vi "Actor Core.vi"(8 "error in":errorcluster, 11 "PW3390 in":refnum<class "PW3390.lvclass">) -> (0 "error out":errorcluster, 3 "Actor out":refnum<class "Actor.lvclass">)   [LabVIEW 2024, in "PW3390 Actor.lvlib" / "PW3390.lvclass"]
doc: "<p>(<strong>Filename</strong>: <span class=\"dnl\">Actor Framework.lvlib:Actor.lvclass:Actor Core.vi</span>)</p>\n<p>Receives messages to the actor, reacts to them, and initiates any error handling that may shut the actor down.</p>\n<p>Descendant classes may override this VI to append parallel tasks for the actor to complete while it handles messages. Overrides use the <a href=\"nihelplauncher://docs/csh?context=lvcore_glang_udclass\">Call Parent Class Method</a> node.</p>"
uses:
  PW3390.lvclass
  C:/Program Files (x86)/National Instruments/LabVIEW 2024/vi.lib/ActorFramework/Actor/Actor.lvclass
  <vilib>/ActorFramework/Actor/Actor.lvclass
  <vilib>/ActorFramework/Actor/Actor.lvclass/Actor.ctl
  PW3390.lvclass/PW3390.ctl
  PW3390Func.ctl
  MFActor/ActorMessage/MF Task Name.ctl
  MFActor/NestedActorName.ctl
  MFActor/DeviceAlias.ctl
  MFActor/ActorMessage/MFActorMsg.lvclass
panel:
  out "Connected":bool
  out "MeasData":dbl[](array[numeric]) format="%.2f"
  out "UpdateData":bool
  out "In Query":bool
  out "connection ID":refnum<k5>
  out "Item":T1(array[cluster])
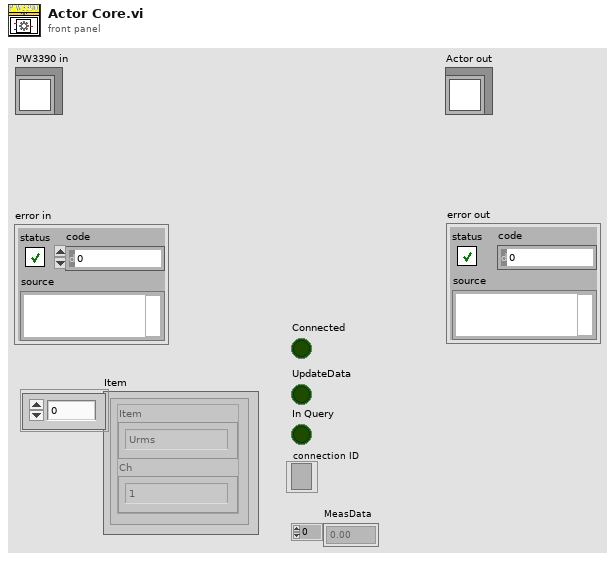
[diagram p1: front panel]
types:
  T1 = cluster{"Item":enum16{"Urms", "Umn", "Uac", "Udc", "Ufnd", "Upk+", "Upk-", "Uthd", "Urf", "Uunb", "Irms", "Imn", "Iac", "Idc", "Ifnd", "Ipk+", "Ipk-", "Ithd", "Irf", "Iunb", "P", "S", "Q", "PF", "DEG U", "DEG I", "DEG P", "f", "EFFI", "LOSS", "IH+", "IH-", "IH", "WP+", "WP-", "WP", "CH A", "CH B", "Pm", "Slip", "TEMP"}, "Ch":enum16{"1", "2", "3", "4", "12", "34", "123"}}[]
  T2 = typedef "PW3390Func.ctl" = enum16{"None", "Wiring", "Config", "Query", "ConvertData", "End"}
  T3 = cluster{"Wiring":u16, "Interface":refnum<visa-resource-name>, "1P Mode":u16, "1P CurrentLimit":dbl, "3P Mode":u16, "3P CurrentLimit":dbl}
  T4 = cluster{"DriverIn":refnum<vi>, "DriverOut":refnum<vi>}
  T5 = cluster{"ManualFetchData":refnum<vi>, "AutoFetchData":refnum<vi>, "SampleRate":refnum<vi>}
  T6 = typedef "NestedActorName.ctl" = enum16{"None", "4503#0", "4503#1", "AIO#0", "AIO#1", "DIO", "PID", "TCPIP", "TestAngle", "TestFixPt", "TestMultiPt", "TestSinWave", "PW3390"}
  T7 = typedef "MF Task Name.ctl" = enum16{"DIChanged", "UpdateErrorCode", "SetTorque", "SetDriveTorque", "DataUpdated", "RunningTestProc", "StreamCtrl", "RunPID", "StopTest", "TCP Conn", "RefreshAutoUI", "ZeroAngle", "NestedActorLaunched", "NestedActorEnded"}
  T8 = typedef "DeviceAlias.ctl" = enum16{"TQM0", "TQM1", "PM", "THERMO", "DC POWER"}
  T9 = cluster{"Data out[0]":dbl, "Data out[1]":dbl, "Data out[2]":dbl, "Data out[3]":dbl, "Data out[4]":dbl, "Data out[5]":dbl, "Data out[6]":dbl, "Data out[7]":dbl, "Data out[8]":dbl, "Data out[9]":dbl}
  T10 = cluster{"Data out[0]":dbl, "Data out[1]":dbl, "Data out[2]":dbl, "Data out[3]":dbl}
  T11 = cluster{"MF Msg Enum":T7, cluster{"MeasData":dbl[], "Device":T8}}
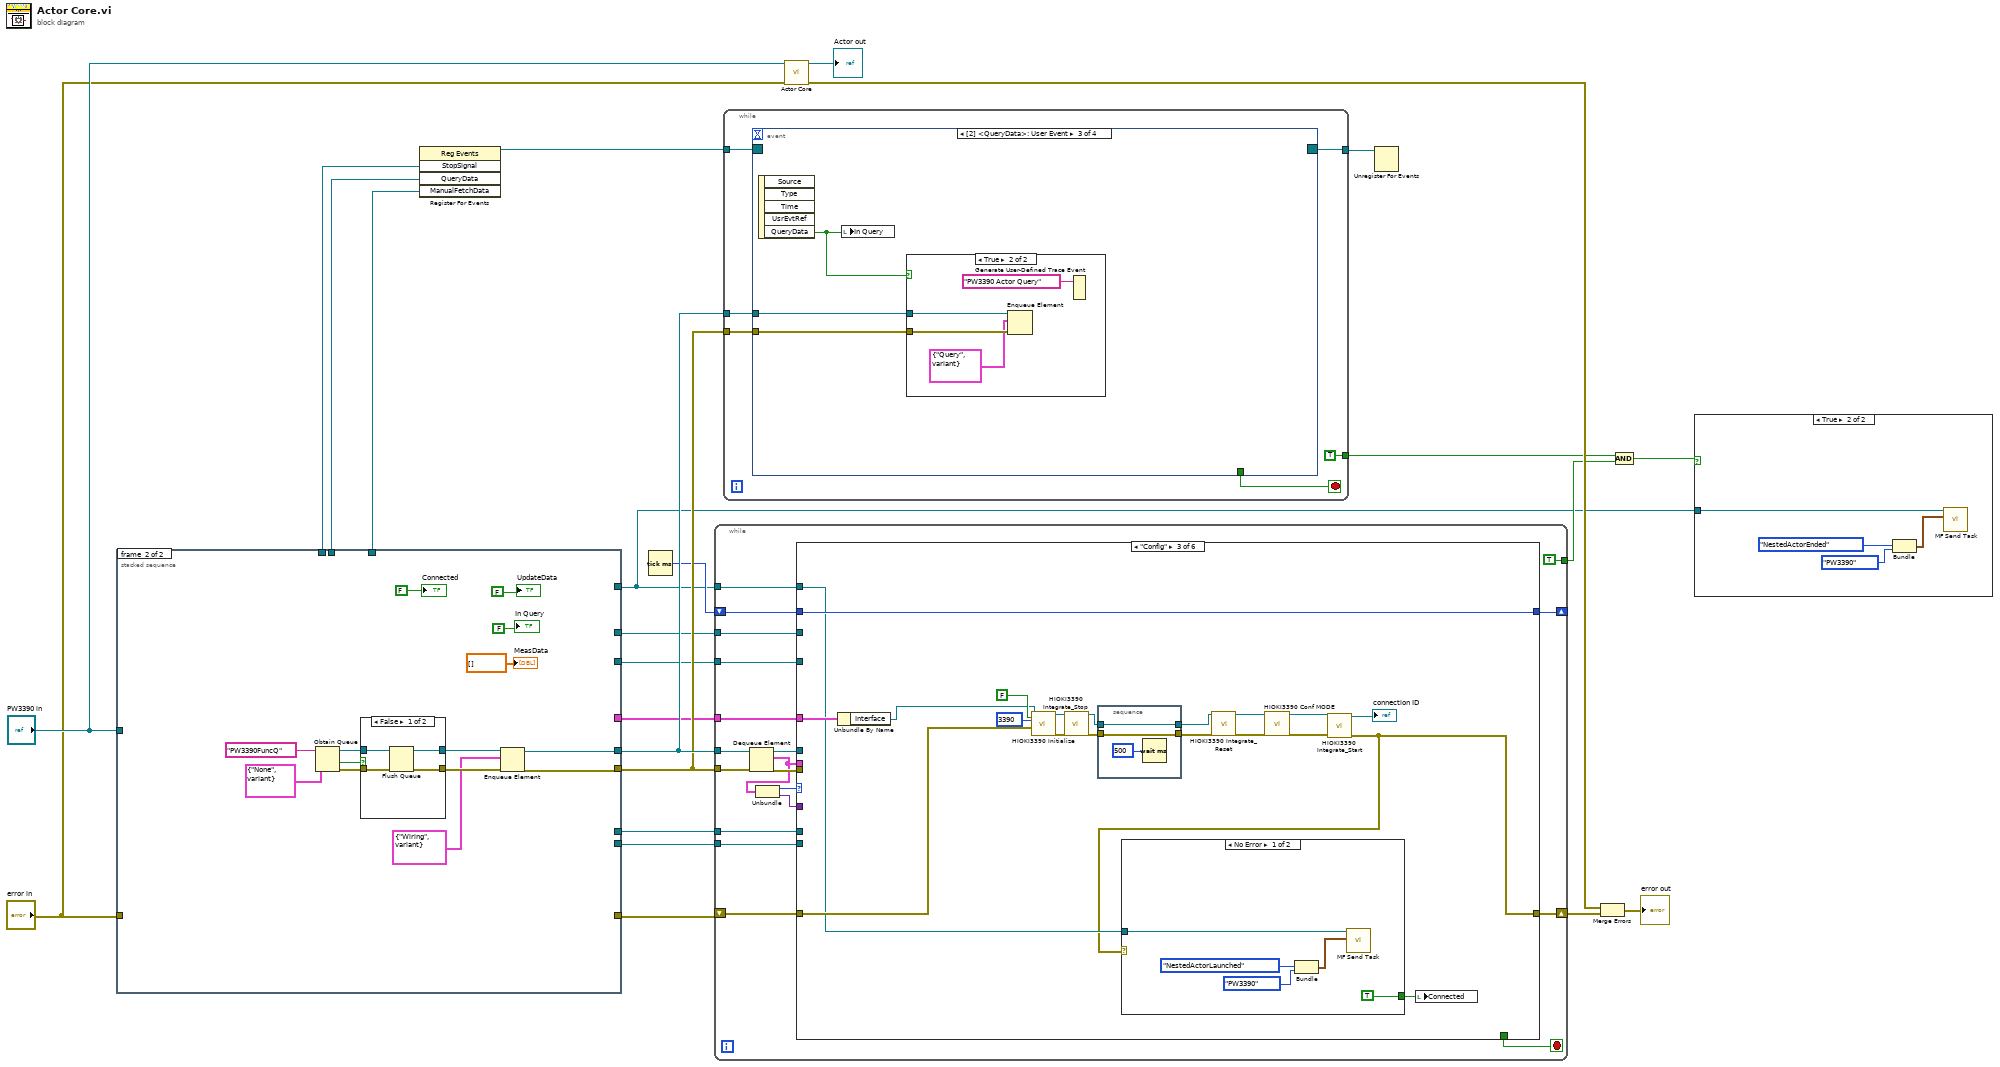
[diagram p0: block diagram]
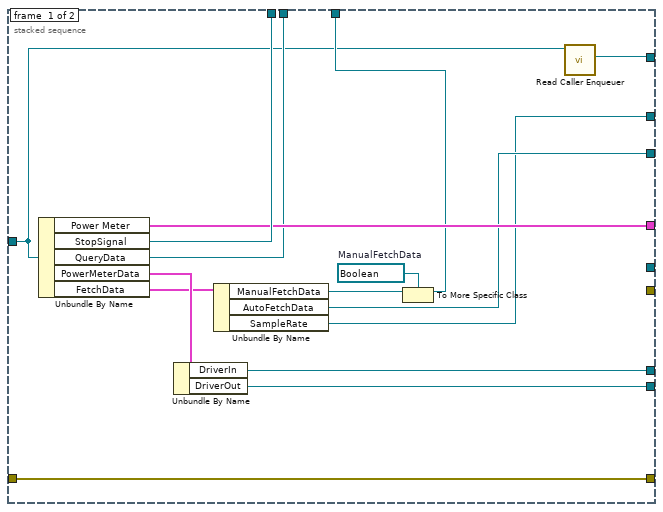
[diagram p3: hidden frame]
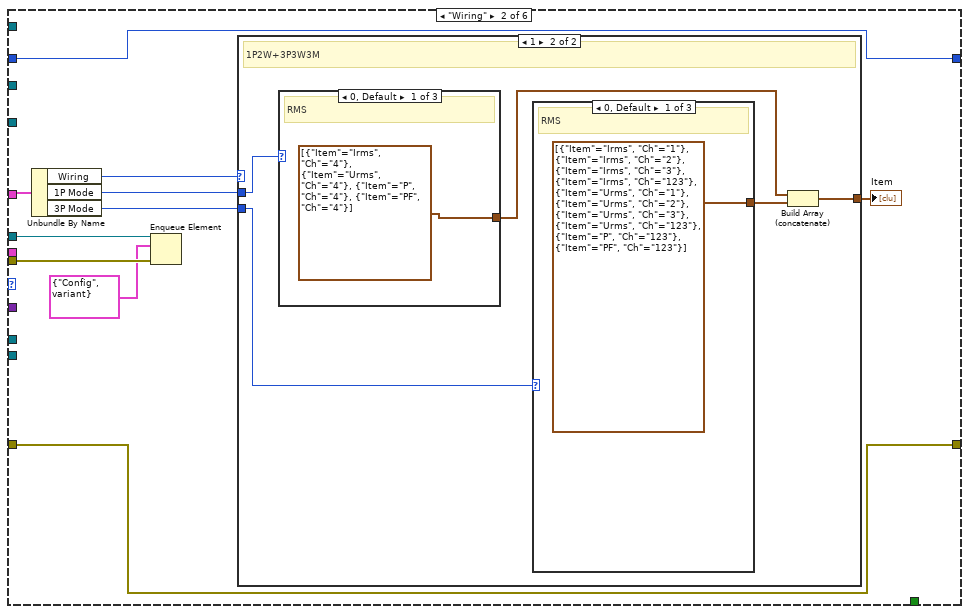
[diagram p6: hidden frame]
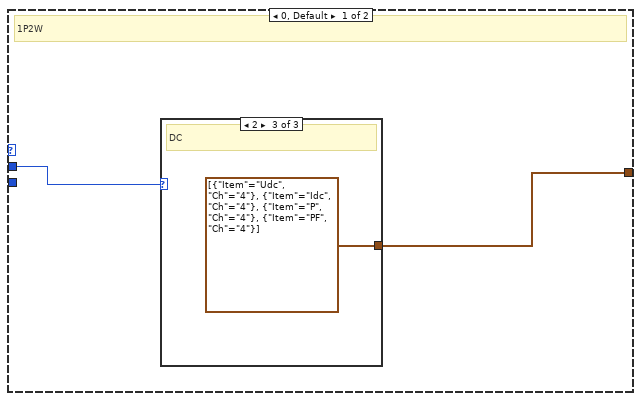
[diagram p7: hidden frame]
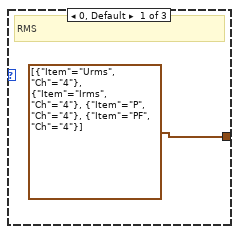
[diagram p8: hidden frame]
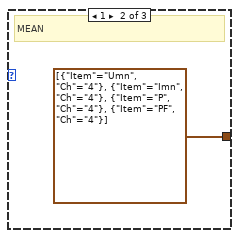
[diagram p9: hidden frame]
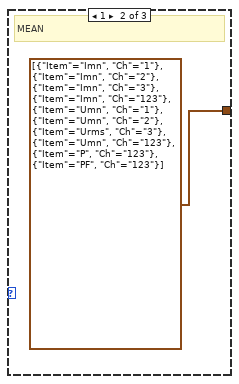
[diagram p10: hidden frame]
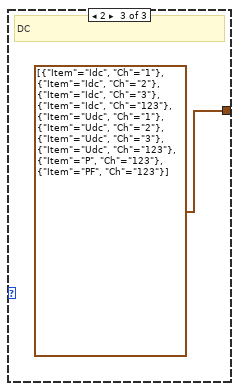
[diagram p11: hidden frame]
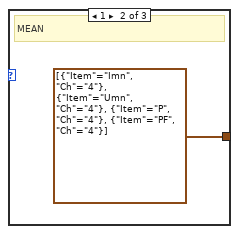
[diagram p12: hidden frame]
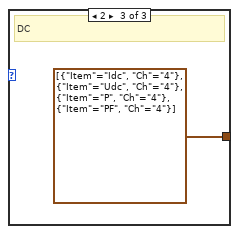
[diagram p13: hidden frame]
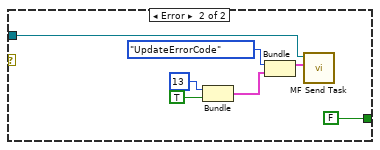
[diagram p14: hidden frame]
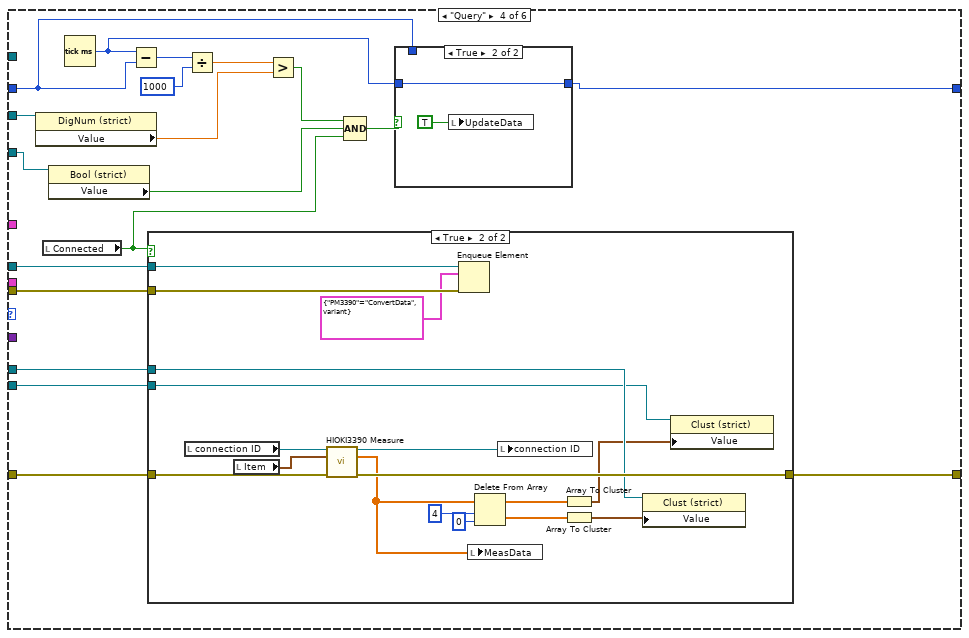
[diagram p15: hidden frame]
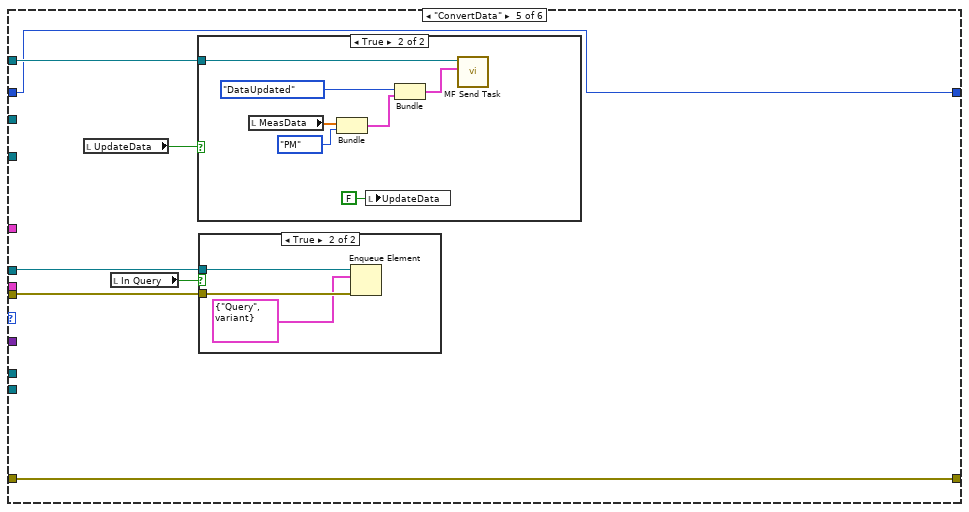
[diagram p18: hidden frame]
diagram:
  n1 = stacked-sequence {
    tunnel: "PW3390 in" -> [w25 _]
    tunnel: [w39 _] -> w23
    tunnel: [_ w45] -> w20
    tunnel: [_ w44] -> w19
    tunnel: [w38 _] -> w18
    tunnel: [w37 _] -> w17
    tunnel: "error in" -> [w37 _]
    tunnel: [w36 _] -> w11
    tunnel: [w34 _] -> w10
    tunnel: [w33 _] -> w9
    tunnel: [w29 _] -> w8
    tunnel: [w28 _] -> w7
    tunnel: [w27 _] -> w6
    tunnel: [w26 _] -> w1
    frame #0 {
      w31 = refnum<vi> refnum  # ManualFetchData
      n2 = Unbundle By Name(w25) -> ("Power Meter"=w38:T3, "StopSignal"=w39:refnum<user-event>, "QueryData"=w36:refnum<user-event>, "PowerMeterData"=w35:T4, "FetchData"=w32:T5)
      n3 = Unbundle By Name(w35) -> ("DriverIn"=w34:refnum<vi>, "DriverOut"=w33:refnum<vi>)
      n4 = Unbundle By Name(w32) -> ("ManualFetchData"=w30:refnum<vi>, "AutoFetchData"=w28:refnum<vi>, "SampleRate"=w27:refnum<vi>)
      n5 = To More Specific Class(target class=w31, reference=w30) -> (specific class reference=w29:refnum<vi>)  [unwired: 1 in, 1 out]
      n6 = call <vilib>:"Read Caller Enqueuer.vi"("Actor"=w25) -> ("Caller Enqueuer"=w26:refnum<class "Message Enqueuer.lvclass">)  [unwired: 10 in]
    }
    frame #1 {
      n7 = Obtain Queue(name (unnamed)="PW3390FuncQ", element data type=cluster{"PM3390":T2, variant} {"PM3390"=enum."None", variant}) -> (queue out=w50:refnum<queue>, created new?=w51:bool, error out=w49:errorcluster)  [unwired: 3 in]
      n8 = case shown="False" w51 {
        tunnel: w50 -> [w57 w59]
        tunnel: w49 -> [w56 w58]
        tunnel: [w55 w59] -> w48
        tunnel: [w54 w58] -> w47
        frame False {
          n9 = Flush Queue(queue=w57, error in (no error)=w56) -> (queue out=w55:refnum<queue>, error out=w54:errorcluster)  [unwired: 1 out]
        }
        frame True {
        }
      }
      n10 = Enqueue Element(queue=w48, element=cluster{"PM3390":T2, variant} {"PM3390"=enum."Wiring", variant}, error in (no error)=w47) -> (queue out=w45:refnum<queue>, error out=w44:errorcluster)  [unwired: 1 in, 1 out]
      "In Query" <- FALSE
      "UpdateData" <- FALSE
      "MeasData" <- dbl[] [] ("MeasData")
      "Connected" <- FALSE
    }
  }
  n11 = register-events(w23, w11, w8) -> (reference out=w12:refnum<event-registration>)  [unwired: 2 in, 1 out]
  n12 = Tick Count (ms)() -> (millisecond timer value=w5:u32)
  n13 = while {
    tunnel: w20 -> [w77]
    tunnel: w19 -> [w78]
    tunnel: w18 -> [w70]
    shift-right: [w68] -> w16
    shift-left: w17 -> [w69]
    tunnel: w10 -> [w67]
    tunnel: w9 -> [w66]
    tunnel: w7 -> [w65]
    tunnel: w6 -> [w64]
    shift-right: [w62] -> _
    shift-left: w5 -> [w63]
    tunnel: w1 -> [w61]
    tunnel: [TRUE] -> w3
    stop <- w71 stop-if-true
    n14 = Dequeue Element(queue=w77, error in (no error)=w78) -> (queue out=w76:refnum<queue>, element=w74:cluster{"PM3390":T2, variant}, error out=w75:errorcluster)  [unwired: 1 in, 1 out]
    n15 = Unbundle(w74) -> ("PM3390"=w73:T2, w72:variant)
    n16 = case shown="\"Config\"" w73 {
      tunnel: w76 -> [_ w85 _ w160 w187 w208]
      tunnel: w75 -> [_ w84 _ w159 w186 w207]
      tunnel: w74 -> [_ _ _ _ _ _]
      tunnel: w72 -> [_ _ _ _ _ _]
      tunnel: [_ _ _ _ _ TRUE] -> w71
      tunnel: w70 -> [_ w90 w126 _ _ _]
      tunnel: w69 -> [w80 w82 w112 w158 w182 w202]
      tunnel: [w80 w82 w108 w157 w182 w201] -> w68
      tunnel: w67 -> [_ _ _ w156 _ _]
      tunnel: w66 -> [_ _ _ w155 _ _]
      tunnel: w65 -> [_ _ _ w150 _ _]
      tunnel: w64 -> [_ _ _ w151 _ _]
      tunnel: w63 -> [w79 w81 w110 w145 w183 w199]
      tunnel: [w79 w81 w110 w143 w183 w199] -> w62
      tunnel: w61 -> [_ _ w109 _ w184 _]
      frame "None", Default {
      }
      frame "Wiring" {
        n17 = Unbundle By Name(w90) -> ("Wiring"=w89:u16, "1P Mode"=w88:u16, "3P Mode"=w87:u16)
        n18 = Enqueue Element(queue=w85, element=cluster{"PM3390":T2, variant} {"PM3390"=enum."Config", variant}, error in (no error)=w84) -> ()  [unwired: 1 in, 3 out]
        n19 = case shown="1" w89 {
          tunnel: w88 -> [w92 w100]
          tunnel: w87 -> [_ w99]
          tunnel: [w91 w96] -> w86
          frame 0, Default {
            # "1P2W"
            n20 = case shown="2" w92 {
              tunnel: [T1 [{"Item"=enum."Urms", "Ch"=enum."4"}, {"Item"=enum."Irms", "Ch"=enum."4"}, {"Item"=enum."P", "Ch"=enum."4"}, {"Item"=enum."PF", "Ch"=enum."4"}] ("Item RMS 2") T1 [{"Item"=enum."Umn", "Ch"=enum."4"}, {"Item"=enum."Imn", "Ch"=enum."4"}, {"Item"=enum."P", "Ch"=enum."4"}, {"Item"=enum."PF", "Ch"=enum."4"}] ("Item RMS 2") T1 [{"Item"=enum."Udc", "Ch"=enum."4"}, {"Item"=enum."Idc", "Ch"=enum."4"}, {"Item"=enum."P", "Ch"=enum."4"}, {"Item"=enum."PF", "Ch"=enum."4"}] ("Item RMS 2")] -> w91
              frame 0, Default {
                # "RMS"
              }
              frame 1 {
                # "MEAN"
              }
              frame 2 {
                # "DC"
              }
            }
          }
          frame 1 {
            # "1P2W+3P3W3M"
            n21 = case shown="0, Default" w100 {
              tunnel: [T1 [{"Item"=enum."Irms", "Ch"=enum."4"}, {"Item"=enum."Urms", "Ch"=enum."4"}, {"Item"=enum."P", "Ch"=enum."4"}, {"Item"=enum."PF", "Ch"=enum."4"}] ("Item RMS 2") T1 [{"Item"=enum."Imn", "Ch"=enum."4"}, {"Item"=enum."Umn", "Ch"=enum."4"}, {"Item"=enum."P", "Ch"=enum."4"}, {"Item"=enum."PF", "Ch"=enum."4"}] ("Item RMS 2") T1 [{"Item"=enum."Idc", "Ch"=enum."4"}, {"Item"=enum."Udc", "Ch"=enum."4"}, {"Item"=enum."P", "Ch"=enum."4"}, {"Item"=enum."PF", "Ch"=enum."4"}] ("Item RMS 2")] -> w98
              frame 0, Default {
                # "RMS"
              }
              frame 1 {
                # "MEAN"
              }
              frame 2 {
                # "DC"
              }
            }
            n22 = case shown="0, Default" w99 {
              tunnel: [T1 [{"Item"=enum."Irms", "Ch"=enum."1"}, {"Item"=enum."Irms", "Ch"=enum."2"}, {"Item"=enum."Irms", "Ch"=enum."3"}, {"Item"=enum."Irms", "Ch"=enum."123"}, {"Item"=enum."Urms", "Ch"=enum."1"}, {"Item"=enum."Urms", "Ch"=enum."2"}, {"Item"=enum."Urms", "Ch"=enum."3"}, {"Item"=enum."Urms", "Ch"=enum."123"}, {"Item"=enum."P", "Ch"=enum."123"}, {"Item"=enum."PF", "Ch"=enum."123"}] ("Item RMS 2") T1 [{"Item"=enum."Imn", "Ch"=enum."1"}, {"Item"=enum."Imn", "Ch"=enum."2"}, {"Item"=enum."Imn", "Ch"=enum."3"}, {"Item"=enum."Imn", "Ch"=enum."123"}, {"Item"=enum."Umn", "Ch"=enum."1"}, {"Item"=enum."Umn", "Ch"=enum."2"}, {"Item"=enum."Urms", "Ch"=enum."3"}, {"Item"=enum."Umn", "Ch"=enum."123"}, {"Item"=enum."P", "Ch"=enum."123"}, {"Item"=enum."PF", "Ch"=enum."123"}] ("Item RMS 2") T1 [{"Item"=enum."Idc", "Ch"=enum."1"}, {"Item"=enum."Idc", "Ch"=enum."2"}, {"Item"=enum."Idc", "Ch"=enum."3"}, {"Item"=enum."Idc", "Ch"=enum."123"}, {"Item"=enum."Udc", "Ch"=enum."1"}, {"Item"=enum."Udc", "Ch"=enum."2"}, {"Item"=enum."Udc", "Ch"=enum."3"}, {"Item"=enum."Udc", "Ch"=enum."123"}, {"Item"=enum."P", "Ch"=enum."123"}, {"Item"=enum."PF", "Ch"=enum."123"}] ("Item RMS 2")] -> w97
              frame 0, Default {
                # "RMS"
              }
              frame 1 {
                # "MEAN"
              }
              frame 2 {
                # "DC"
              }
            }
            n23 = Build Array (concatenate)(w98, w97) -> (w96:T1)
          }
        }
        "Item" <- w86
      }
      frame "Config" {
        n24 = Unbundle By Name(w126) -> ("Interface"=w115:refnum<visa-resource-name>)
        n25 = call "HIOKI3390 Initialize.vi"("Address"=w115, "Reset (T:Yes)"=FALSE, "Port"=u16 3390, "error in (no error)"=w112) -> ("connection ID out"=w123:refnum<k5>, "error out"=w124:errorcluster)  [unwired: 9 in, 1 out]
        n26 = call "HIOKI3390 Integrate_Stop.vi"("connection ID"=w123, "error in (no error)"=w124) -> ("connection ID out"=w122:refnum<k5>, "error out"=w121:errorcluster)  [unwired: 12 in]
        n27 = stacked-sequence {
          tunnel: [w139] -> w120
          tunnel: w122 -> [w139]
          tunnel: w121 -> [w140]
          tunnel: [w140] -> w119
          frame #0 {
            n28 = Wait (ms)(milliseconds to wait=u32 500 ("ミリ秒待ち時間")) -> ()  [unwired: 1 out]
          }
        }
        n29 = call "HIOKI3390 Integrate_Reset.vi"("connection ID"=w120, "error in (no error)"=w119) -> ("connection ID out"=w117:refnum<k5>, "error out"=w118:errorcluster)  [unwired: 12 in]
        n30 = call "HIOKI3390 Conf MODE.vi"("connection ID"=w117, "error in (no error)"=w118) -> ("connection ID out"=w114:refnum<k5>, "error out"=w113:errorcluster)  [unwired: 11 in, 1 out]
        n31 = call "HIOKI3390 Integrate_Start.vi"("connection ID"=w114, "error in (no error)"=w113) -> ("connection ID out"=→"connection ID":refnum<k5>, "error out"=w108:errorcluster)  [unwired: 12 in]
        n32 = case shown="No Error" w108 {
          tunnel: w109 -> [w130 w133]
          tunnel: [TRUE FALSE] -> w107
          frame No Error {
            n33 = Bundle("MF Msg Enum"=MF_Task_Name."NestedActorLaunched", "NestedActorName"=NestedActorName."PW3390") -> (w127:cluster{"MF Msg Enum":T7, "NestedActorName":T6})  [unwired: 1 in]
            n34 = call "MF Send Task.vi"("MsgType"=w127, "Message Enqueuer"=w130) -> ()  [unwired: 9 in, 1 out]
          }
          frame Error {
            n35 = Bundle(13, TRUE) -> (w135:cluster{i32, bool})  [unwired: 1 in]
            n36 = Bundle("MF Msg Enum"=MF_Task_Name."UpdateErrorCode", w135) -> (w138:cluster{"MF Msg Enum":T7, cluster{i32, bool}})  [unwired: 1 in]
            n37 = call "MF Send Task.vi"("MsgType"=w138, "Message Enqueuer"=w133) -> ()  [unwired: 9 in, 1 out]
          }
        }
        n38 = local write "Connected"(w107) -> ()
      }
      frame "Query" {
        n39 = property class="DigNum (strict)"(reference=w151) -> ("Value"=w149:dbl)  [unwired: 1 in, 2 out]
        n40 = local read "Connected"() -> (w142:bool)
        n41 = property class="Bool (strict)"(reference=w150) -> ("Value"=w147:bool)  [unwired: 1 in, 2 out]
        n42 = Tick Count (ms)() -> (millisecond timer value=w144:u32)
        n43 = Subtract(x=w144, y=w145) -> (x-y=w154:u32)
        n44 = case shown="True" w142 {
          tunnel: w160 -> [_ w178]
          tunnel: w159 -> [_ w177]
          tunnel: w158 -> [w161 w174]
          tunnel: [w161 w172] -> w157
          tunnel: w156 -> [_ w169]
          tunnel: w155 -> [_ w166]
          frame False {
          }
          frame True {
            n45 = local read "connection ID"() -> (w176:refnum<k5>)
            n46 = local read "Item"() -> (w175:T1)
            n47 = call "HIOKI3390 Measure.vi"("connection ID"=w176, "Item"=w175, "error in (no error)"=w174) -> ("connection ID"=w173:refnum<k5>, "Data out"=w162:dbl[], "error out"=w172:errorcluster)  [unwired: 8 in, 2 out]
            n48 = Enqueue Element(queue=w178, element=cluster{"PM3390":T2, variant} {"PM3390"=enum."ConvertData", variant}, error in (no error)=w177) -> ()  [unwired: 1 in, 3 out]
            n49 = local write "MeasData"(w162) -> ()
            n50 = Delete From Array(array=w162, length=4, index=0) -> (deleted portion=w168:dbl[], array with subset deleted=w165:dbl[])
            n51 = local write "connection ID"(w173) -> ()
            n52 = Array To Cluster(array=w165) -> (cluster=w164:T9)
            n53 = Array To Cluster(array=w168) -> (cluster=w167:T10)
            n54 = property class="Clust (strict)"(reference=w169, "Value"=w167) -> ()  [unwired: 1 in, 2 out]
            n55 = property class="Clust (strict)"(reference=w166, "Value"=w164) -> ()  [unwired: 1 in, 2 out]
          }
        }
        n56 = Divide(x=w154, y=u32 1000) -> (x/y=w152:dbl)
        n57 = Greater?(x=w152, y=w149) -> (0:w148:bool)
        n58 = Compound Arithmetic op=AND(w148, w147, w142) -> (w146:bool)
        n59 = case shown="True" w146 {
          tunnel: w145 -> [w179 _]
          tunnel: w144 -> [_ w180]
          tunnel: [w179 w180] -> w143
          frame False {
          }
          frame True {
            n60 = local write "UpdateData"(TRUE) -> ()
          }
        }
      }
      frame "ConvertData" {
        n61 = local read "UpdateData"() -> (w185:bool)
        n62 = local read "In Query"() -> (w188:bool)
        n63 = case shown="True" w185 {
          tunnel: w184 -> [_ w194]
          frame False {
          }
          frame True {
            n64 = local read "MeasData"() -> (w193:dbl[])
            n65 = Bundle("MeasData"=w193, "Device"=DeviceAlias."PM") -> (w190:cluster{"MeasData":dbl[], "Device":T8})  [unwired: 1 in]
            n66 = local write "UpdateData"(FALSE ("UpdateData")) -> ()
            n67 = Bundle("MF Msg Enum"=MF_Task_Name."DataUpdated", w190) -> (w189:T11)  [unwired: 1 in]
            n68 = call "MF Send Task.vi"("MsgType"=w189, "Message Enqueuer"=w194) -> ()  [unwired: 9 in, 1 out]
          }
        }
        n69 = case shown="True" w188 {
          tunnel: w187 -> [_ w198]
          tunnel: w186 -> [_ w197]
          frame False {
          }
          frame True {
            n70 = Enqueue Element(queue=w198, element=cluster{"PM3390":T2, variant} {"PM3390"=enum."Query", variant}, error in (no error)=w197) -> ()  [unwired: 1 in, 3 out]
          }
        }
      }
      frame "End" {
        n71 = Flush Queue(queue=w208, error in (no error)=w207) -> (queue out=w206:refnum<queue>, error out=w205:errorcluster)  [unwired: 1 out]
        n72 = Release Queue(queue=w206, error in (no error)=w205) -> ()  [unwired: 1 in, 3 out]
        n73 = local read "connection ID"() -> (w203:refnum<k5>)
        n74 = call "HIOKI3390 Close.vi"("connection ID"=w203, "error in (no error)"=w202) -> ("error out"=w201:errorcluster)  [unwired: 13 in]
        n75 = Generate User-Defined Trace Event(2:"PW3390 Actor End" ("trace string")) -> ()  [unwired: 1 in]
      }
    }
  }
  n76 = while {
    tunnel: [w214] -> w22
    tunnel: w20 -> [w213]
    tunnel: w19 -> [w212]
    tunnel: w12 -> [w210]
    tunnel: [TRUE] -> w4
    stop <- w211 stop-if-true
    n77 = event shown="[2] <QueryData>: User Event" {
      selector: w210 -> [_ _ _ _]
      dyn-events: [_ _ _ _] -> w214
      timeout: _ -> [_ _ _ _]
      tunnel: w213 -> [_ w219 w225 _]
      tunnel: w212 -> [_ w218 w224 _]
      tunnel: [_ TRUE _ _] -> w211
      event Timeout {
        n78 = event-data() -> ()  [unwired: 1 in, 3 out]
      }
      event User Event {
        n79 = event-data() -> ()  [unwired: 1 in, 5 out]
        n80 = Flush Queue(queue=w219, error in (no error)=w218) -> (queue out=w217:refnum<queue>, error out=w216:errorcluster)  [unwired: 1 out]
        n81 = local write "In Query"(FALSE ("In Query")) -> ()
        n82 = local write "UpdateData"(FALSE ("UpdateData")) -> ()
        n83 = Enqueue Element At Opposite End(queue=w217, element=cluster{"PM3390":T2, variant} {"PM3390"=enum."End", variant}, error in (no error)=w216) -> ()  [unwired: 1 in, 3 out]
        n84 = local write "Connected"(FALSE) -> ()
      }
      event User Event {
        n85 = event-data() -> ("QueryData"=w226:bool)  [unwired: 1 in, 4 out]
        n86 = local write "In Query"(w226) -> ()
        n87 = case shown="True" w226 {
          tunnel: w225 -> [_ w230]
          tunnel: w224 -> [_ w229]
          frame False {
          }
          frame True {
            n88 = Enqueue Element(queue=w230, element=cluster{"PM3390":T2, variant} {"PM3390"=enum."Query", variant}, error in (no error)=w229) -> ()  [unwired: 1 in, 3 out]
            n89 = Generate User-Defined Trace Event(2:"PW3390 Actor Query" ("trace string")) -> ()  [unwired: 1 in]
          }
        }
      }
      event Value Change {
        n90 = event-data() -> ()  [unwired: 1 in, 6 out]
        n91 = local write "UpdateData"(TRUE) -> ()
      }
    }
  }
  n92 = call-parent "Actor Core.vi"("error in"="error in", "Actor in"="PW3390 in") -> ("error out"=w14:errorcluster, "Actor out"=→"Actor out":refnum<class "Actor.lvclass">)  [unwired: 8 in]
  n93 = Unregister For Events(event registration refnum=w22) -> ()  [unwired: 1 in, 1 out]
  n94 = Merge Errors(w14, w16) -> (→"error out":errorcluster)
  n95 = Compound Arithmetic op=AND(w4, w3) -> (w2:bool)
  n96 = case shown="True" w2 {
    tunnel: w1 -> [_ w232]
    frame False {
    }
    frame True {
      n97 = Bundle("MF Msg Enum"=MF_Task_Name."NestedActorEnded", "NestedActorName"=NestedActorName."PW3390") -> (w235:cluster{"MF Msg Enum":T7, "NestedActorName":T6})  [unwired: 1 in]
      n98 = call "MF Send Task.vi"("MsgType"=w235, "Message Enqueuer"=w232) -> ()  [unwired: 9 in, 1 out]
    }
  }
